vi "run_simulation_backup.vi"(4 "Output File Loaded?":refnum<vi>, 7 "Spec File Loaded":bool, 9 "Run":refnum<vi>, 10 "Numeric":i32, 11 "Parameters":refnum<vi>) -> (0 "OK":bool, 1 "TMP Filepath":path, 2 "standard error":string, 3 "standard output":string)   [LabVIEW 2019]
uses:
  <vilib>/Utility/sysdir.llb/System Directory Type.ctl
  LUATableParser/libLUATableReader.so
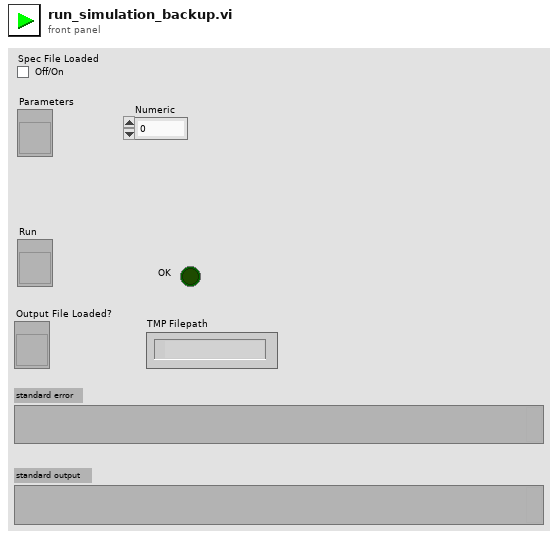
[diagram p1: front panel]
types:
  T1 = enum8{"Enabled", "Disabled", "Disabled and Grayed Out"}
  T2 = typedef "System Directory Type.ctl" = i32
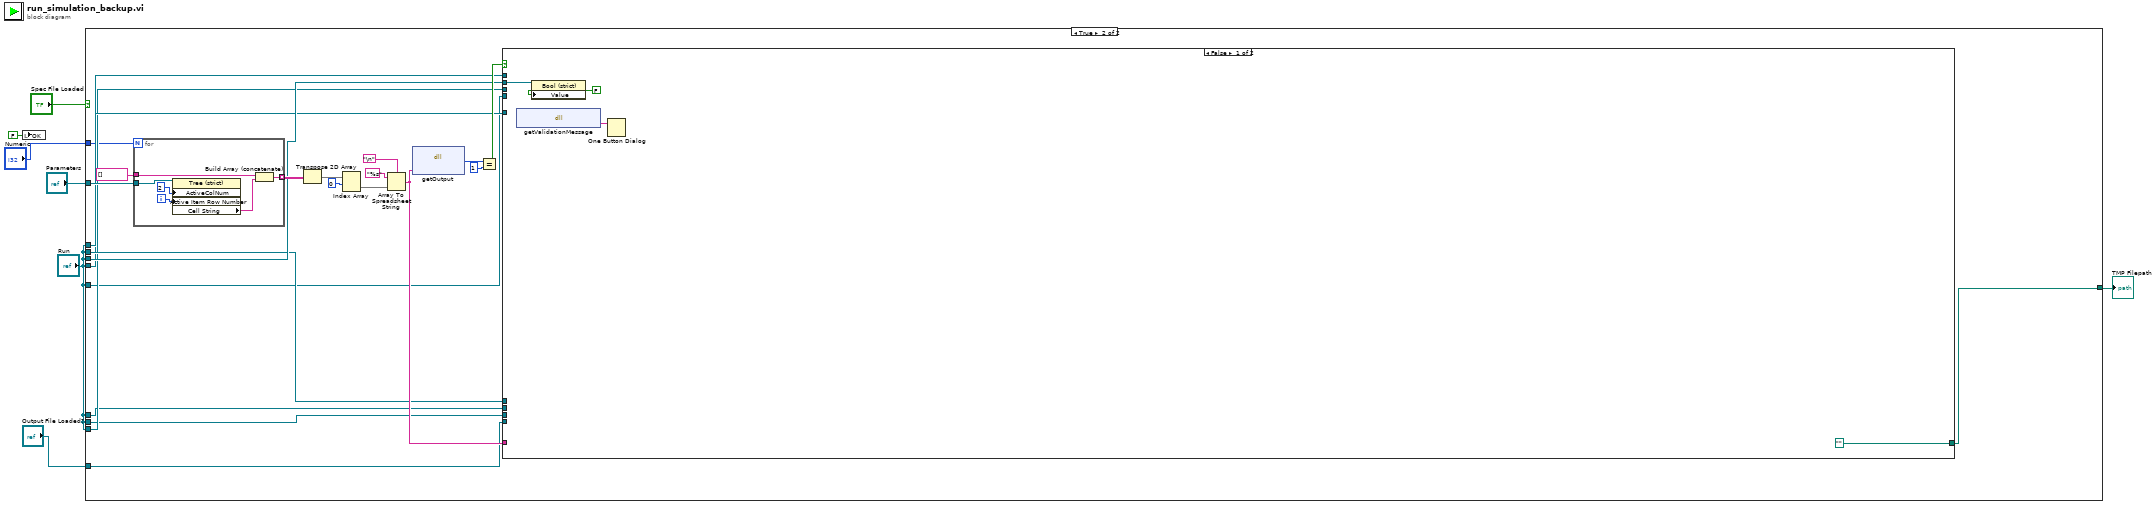
[diagram p0: block diagram]
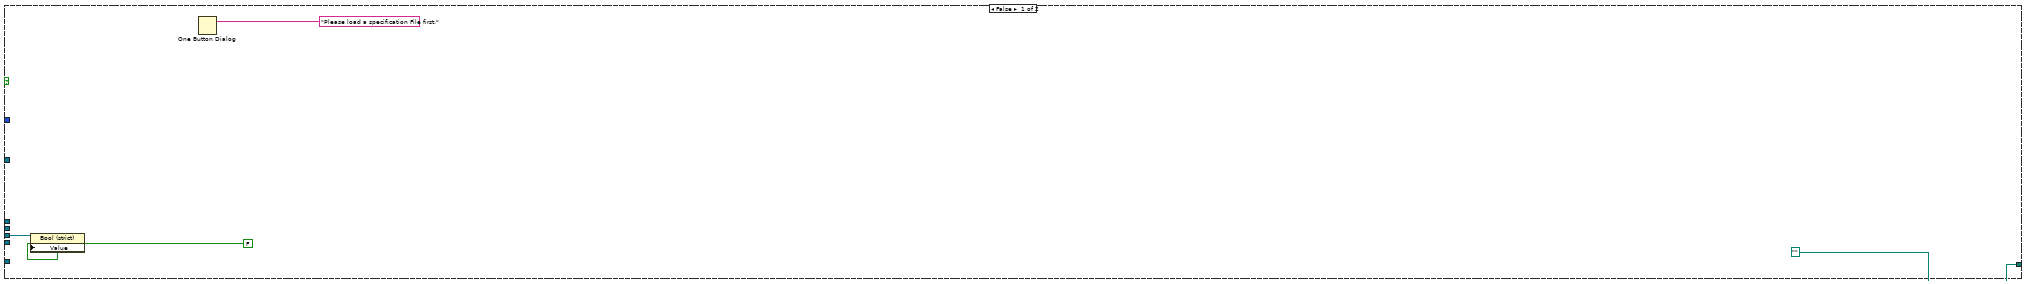
[diagram p2: hidden frame]
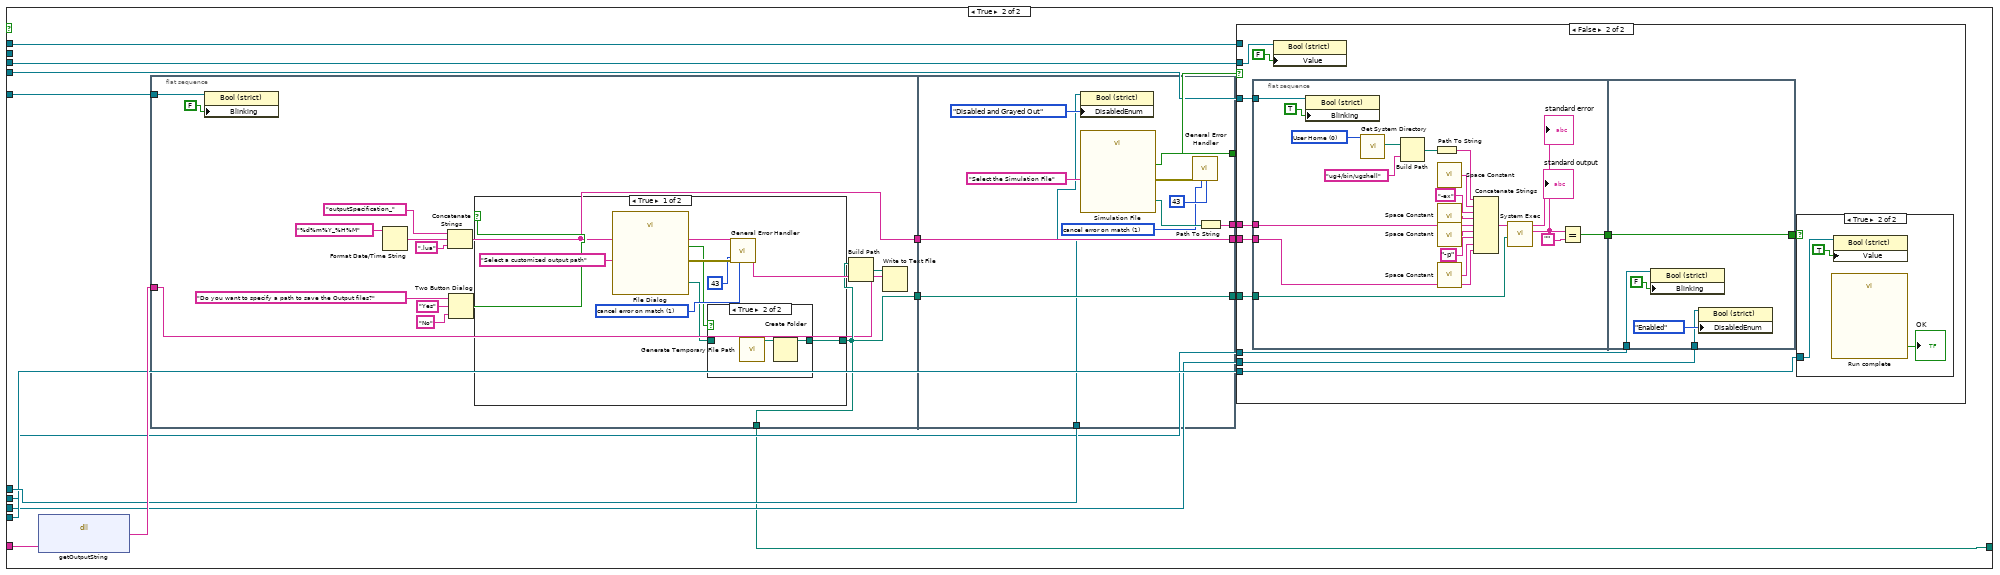
[diagram p3: hidden frame]
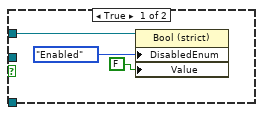
[diagram p4: hidden frame]
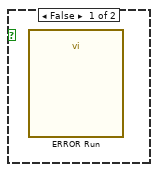
[diagram p5: hidden frame]
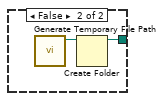
[diagram p7: hidden frame]
diagram:
  n1 = local write "OK"(FALSE ("OK")) -> ()
  n2 = case shown="True" "Spec File Loaded" {
    tunnel: "Parameters" -> [_ w23]
    tunnel: "Run" -> [w9 w22]
    tunnel: "Run" -> [_ w21]
    tunnel: "Run" -> [_ w20]
    tunnel: "Run" -> [_ w19]
    tunnel: "Output File Loaded?" -> [_ w18]
    tunnel: "Run" -> [_ w17]
    tunnel: "Run" -> [_ w16]
    tunnel: "Run" -> [_ w15]
    tunnel: "Run" -> [_ w14]
    tunnel: [path "" w13] -> w3
    tunnel: "Numeric" -> [_ w12]
    frame False {
      n3 = property on="Property Node" class="Bool (strict)"(reference=w9, "Value"=FALSE) -> ()  [unwired: 1 in, 2 out]
      n4 = One Button Dialog(message="Please load a specification File first.") -> ()  [unwired: 1 in, 1 out]
    }
    frame True {
      n5 = for {
        N: w12 -> [_]
        tunnel: string[] [] ("Empty Val Arr") -> [w139]
        tunnel: [w138] -> w33 mode=indexing
        tunnel: w23 -> [w136]
        i -> [w141]
        n6 = property on="Property Node" class="Tree (strict)"(reference=w136, "ActiveColNum"=2 ("Active Cell:Active Column Number"), "Active Item Row Number"=w141) -> ("Cell String"=w137:string)  [unwired: 1 in, 2 out]
        n7 = Build Array (concatenate)(w139, w137) -> (w138:string[])
      }
      n8 = Transpose 2D Array(2D array=w33) -> (transposed array=w32:string[][])
      n9 = Index Array(array=w32, index (row)=0) -> (element=w31:string[])  [unwired: 1 in]
      n10 = Array To Spreadsheet String(delimiter (Tab)="\n", array=w31, 3:"%s" ("format string")) -> (spreadsheet string=w24:string)
      n11 = dll-call lib="home/paul/Schreibtisch/LUATableParser/libLUATableReader.so" fn="getOutput"("inputSpecs"=w24) -> ("isValid"=w25:i32)  [unwired: 4 in, 2 out]
      n12 = Equal?(x=w25, y=1) -> (x = y?=w27:bool)
      n13 = case shown="False" w27 {
        tunnel: w24 -> [_ w55]
        tunnel: w22 -> [w36 _]
        tunnel: w21 -> [_ w49]
        tunnel: w20 -> [_ w48]
        tunnel: w19 -> [_ w47]
        tunnel: w18 -> [_ w46]
        tunnel: w17 -> [_ w45]
        tunnel: w16 -> [_ w44]
        tunnel: w15 -> [_ w43]
        tunnel: w14 -> [_ w42]
        tunnel: [path "" w41] -> w13
        frame False {
          n14 = dll-call lib="home/paul/Schreibtisch/LUATableParser/libLUATableReader.so" fn="getValidationMessage"() -> ("validationMessage"=w38:string)  [unwired: 3 in, 2 out]
          n15 = property on="Property Node" class="Bool (strict)"(reference=w36, "Value"=FALSE ("Run")) -> ()  [unwired: 1 in, 2 out]
          n16 = One Button Dialog(message=w38) -> ()  [unwired: 1 in, 1 out]
        }
        frame True {
          n17 = dll-call lib="home/paul/Schreibtisch/LUATableParser/libLUATableReader.so" fn="getOutputString"("inputSpecs"=w55) -> ("outputString"=w54:string)  [unwired: 4 in, 2 out]
          n18 = flat-sequence {
            tunnel: w54 -> [w99]
            tunnel: [w100] -> w40
            tunnel: [w102] -> w39
            tunnel: w49 -> [w111]
            tunnel: [w100] -> w41
            tunnel: w40 -> [w128]
            tunnel: w39 -> [w129]
            tunnel: [w130] -> w53
            tunnel: [w129] -> w52
            tunnel: [w128] -> w51
            tunnel: [w127] -> w50
            tunnel: w48 -> [w125]
            frame #0 {
              n19 = property on="Property Node" class="Bool (strict)"(reference=w111, "Blinking"=FALSE) -> ()  [unwired: 1 in, 2 out]
              n20 = Format Date/Time String(time format string (%c)="%d%m%Y_%H%M") -> (date/time string=w104:string)  [unwired: 2 in]
              n21 = Concatenate Strings("outputSpecification_" ("string"), w104, ".lua" ("string")) -> (w102:string)
              n22 = Two Button Dialog(message="Do you want to specify a path to save the Output files?", 1:"No" ("F button name (\"Cancel\")"), 2:"Yes" ("T button name (\"OK\")")) -> (T button?=w107:bool)
              n23 = case shown="True" w107 {
                tunnel: [w115 w123] -> w100
                frame True {
                  w117 = 1 items=["no exception", "cancel error on match", "set error on match"] ("[exception action] (none:0)")
                  n24 = call "File Dialog"("prompt"="Select a customized output path") -> ("selected path"=w116:path, "cancelled"=w114:bool, "error out"=w119:errorcluster)  [unwired: 11 in, 1 out]
                  n25 = case shown="True" w114 {
                    tunnel: w116 -> [w120 _]
                    tunnel: [w120 w121] -> w115
                    frame False {
                    }
                    frame True {
                      n26 = call <vilib>:"Generate Temporary File Path.vi"() -> ("Unique Temporary File Path"=w122:path)  [unwired: 10 in, 1 out]
                      n27 = Create Folder(path (use dialog)=w122) -> (created path=w121:path)  [unwired: 2 in, 2 out]
                    }
                  }
                  n28 = call <vilib>:"General Error Handler.vi"("error in (no error)"=w119, "[exception action] (none:0)"=w117, "[exception code]"=43) -> ()  [unwired: 8 in, 5 out]
                }
                frame False {
                  n29 = call <vilib>:"Generate Temporary File Path.vi"() -> ("Unique Temporary File Path"=w124:path)  [unwired: 10 in, 1 out]
                  n30 = Create Folder(path (use dialog)=w124) -> (created path=w123:path)  [unwired: 2 in, 2 out]
                }
              }
              n31 = Build Path(base path=w100, name or relative path=w102) -> (appended path=w101:path)
              n32 = Write to Text File(file (use dialog)=w101, text=w99) -> ()  [unwired: 2 in, 3 out]
            }
            frame #1 {
              w132 = 1 items=["no exception", "cancel error on match", "set error on match"] ("[exception action] (none:0)")
              n33 = property on="Property Node" class="Bool (strict)"(reference=w125, "DisabledEnum"=T1."Disabled and Grayed Out" ("Disabled")) -> ()  [unwired: 1 in, 2 out]
              n34 = call "Simulation File"("prompt"="Select the Simulation File") -> ("selected path"=w134:path, "cancelled"=w130:bool, "error out"=w131:errorcluster)  [unwired: 11 in, 1 out]
              n35 = call <vilib>:"General Error Handler.vi"("error in (no error)"=w131, "[exception action] (none:0)"=w132, "[exception code]"=43) -> ()  [unwired: 8 in, 5 out]
              n36 = Path To String(path=w134) -> (string=w127:string)
            }
          }
          n37 = case shown="False" w53 {
            tunnel: w52 -> [_ w67]
            tunnel: w51 -> [_ w68]
            tunnel: w50 -> [_ w66]
            tunnel: w47 -> [w57 _]
            tunnel: w46 -> [_ w63]
            tunnel: w45 -> [_ w62]
            tunnel: w44 -> [_ w61]
            tunnel: w43 -> [_ w60]
            tunnel: w42 -> [_ w59]
            frame True {
              n38 = property on="Property Node" class="Bool (strict)"(reference=w57, "DisabledEnum"=T1."Enabled" ("Disabled"), "Value"=FALSE) -> ()  [unwired: 1 in, 2 out]
            }
            frame False {
              n39 = flat-sequence {
                tunnel: w68 -> [w77]
                tunnel: w67 -> [w76]
                tunnel: w66 -> [w75]
                tunnel: [w72] -> w64
                tunnel: w61 -> [w71]
                tunnel: [w95] -> w65
                tunnel: w64 -> [w95]
                tunnel: w60 -> [w92]
                tunnel: w59 -> [w91]
                frame #0 {
                  w81 = T2 0 items=["User Home"=0, "User Desktop"=1, "User Documents"=2, "User Application Data"=3, "User Preferences"=4, "User Temporary"=5, "Public Documents"=6, "Public Application Data"=7, "Public Preferences"=8, "Public Cache"=13, "System Core Libraries"=9, "System Installed Libraries"=10, "Application Files"=11, "Boot Volume Root"=12] ("system directory type")
                  n40 = property on="Property Node" class="Bool (strict)"(reference=w71, "Blinking"=TRUE) -> ()  [unwired: 1 in, 2 out]
                  n41 = call <vilib>:"Get System Directory.vi"("system directory type"=w81) -> ("system directory"=w89:path)  [unwired: 10 in]
                  n42 = Build Path(base path=w89, name or relative path="ug4/bin/ugshell") -> (appended path=w87:path)
                  n43 = Path To String(path=w87) -> (string=w83:string)
                  n44 = call <vilib>:"Space Constant.vi"() -> ("String"=w84:string)
                  n45 = call <vilib>:"Space Constant.vi"() -> ("String"=w85:string)
                  n46 = call <vilib>:"Space Constant.vi"() -> ("String"=w86:string)
                  n47 = call <vilib>:"Space Constant.vi"() -> ("String"=w90:string)
                  n48 = Concatenate Strings(w83, w84, "-ex" ("command line"), w85, w75, w86, "-p" ("command line"), w90, w76) -> (w88:string)
                  n49 = call <vilib>:"System Exec.vi"("working directory"=w77, "command line"=w88) -> ("standard error"=w73:string, "standard output"=→"standard output":string)  [unwired: 6 in, 2 out]
                  "standard error" <- w73
                  n50 = Equal?(x=w73, y="") -> (x = y?=w72:bool)
                }
                frame #1 {
                  n51 = property on="Property Node" class="Bool (strict)"(reference=w91, "Blinking"=FALSE) -> ()  [unwired: 1 in, 2 out]
                  n52 = property on="Property Node" class="Bool (strict)"(reference=w92, "DisabledEnum"=T1."Enabled" ("Disabled")) -> ()  [unwired: 1 in, 2 out]
                }
              }
              n53 = property class="Bool (strict)"(reference=w62, "Value"=FALSE ("Run")) -> ()  [unwired: 1 in, 2 out]
              n54 = case shown="True" w65 {
                tunnel: w63 -> [_ w97]
                frame False {
                  n55 = call "ERROR Run"() -> ()  [unwired: 10 in, 2 out]
                }
                frame True {
                  n56 = call "Run complete"() -> ("OK"=→"OK":bool)  [unwired: 10 in, 1 out]
                  n57 = property class="Bool (strict)"(reference=w97, "Value"=TRUE ("Succesfull Run")) -> ()  [unwired: 1 in, 2 out]
                }
              }
            }
          }
        }
      }
    }
  }
  "TMP Filepath" <- w3
